vi "PutMotorPower.vi"(8 "ErrorIn(no error)":errorcluster, 10 "MotorPower":T1, 11 "FPGA VI引用输入":refnum<k20>) -> (0 "ErrorOut":errorcluster, 3 "FPGA VI引用输出":refnum<k20>)   [LabVIEW 2015]
uses:
  <vilib>/Utility/error.llb/Error Cluster From Error Code.vi
  <vilib>/rvi/errors/niLvFpgaAdjustHostInterfaceError.vi
  <vilib>/rvi/interface/nirviReadWriteControl/nirviReadWriteControl.xnode
  NiFpgaLv.dll
  <vilib>/rvi/interface/Simulation/niFpgaSimulationCallBeginRW.vi
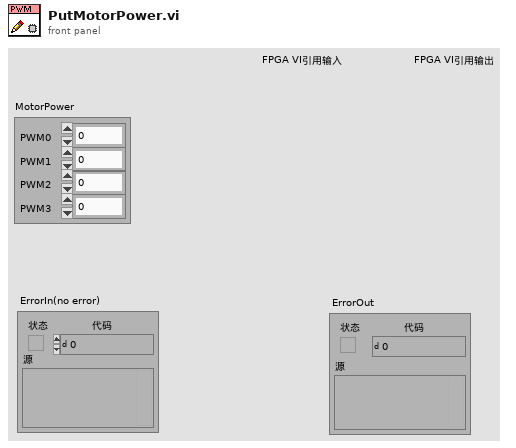
[diagram p1: front panel]
types:
  T1 = cluster{"PWM0":u16, "PWM1":u16, "PWM2":u16, "PWM3":u16}
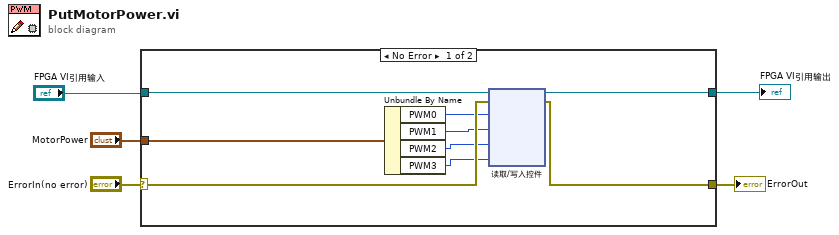
[diagram p0: block diagram]
diagram:
  n1 = case shown="No Error" "ErrorIn(no error)" {
    selector: "ErrorIn(no error)" -> [w13 w15]
    tunnel: "FPGA VI引用输入" -> [w14 w16]
    tunnel: [w12 w16] -> w1
    tunnel: [w11 w15] -> w4
    tunnel: "MotorPower" -> [w10 _]
    frame No Error {
      n2 = Unbundle By Name(w10) -> ("PWM0"=w9:u16, "PWM1"=w8:u16, "PWM2"=w7:u16, "PWM3"=w6:u16)
      n3 = xnode "读取/写入控件"("FPGA VI Reference In"=w14, "error in"=w13, "PWM0"=w9, "PWM1"=w8, "PWM2"=w7, "PWM3"=w6) -> ("FPGA VI Reference Out"=w12:refnum<k20>, "error out"=w11:errorcluster)
    }
    frame Error {
    }
  }
  "ErrorOut" <- w4
  "FPGA VI引用输出" <- w1
